vi "Smooth Volume.vi"(4 "Trigger":bool, 8 "Volume In":dbl format="%#_13g") -> (0 "Volume Out":sgl)   [LabVIEW 2015]
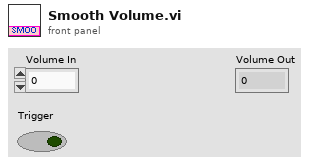
[diagram p1: front panel]
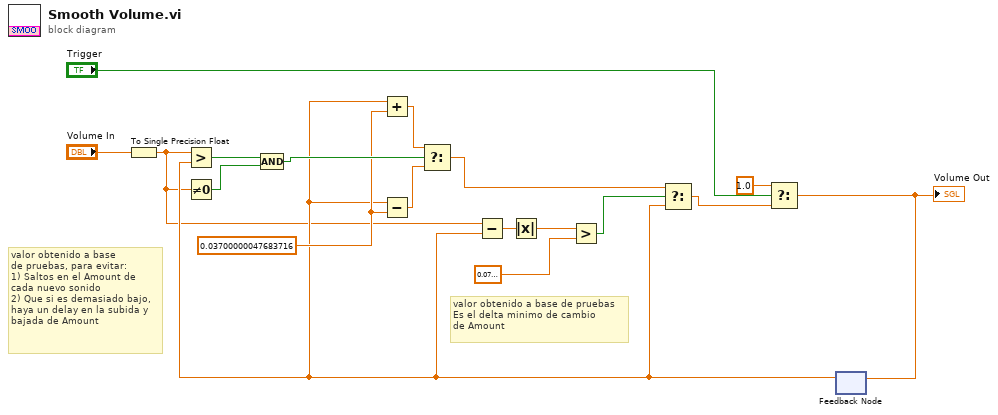
[diagram p0: block diagram]
diagram:
  w13 = sgl 0.037 ("factor")
  # "valor obtenido a base de pruebas\nEs el delta minimo de cambio\nde Amount"
  # "valor obtenido a base\nde pruebas, para evitar:\n1) Saltos en el Amount de\ncada nuevo sonido\n2) Que si es demasiado bajo,\nhaya un delay en la subida y\nbajada de Amount"
  n1 = To Single Precision Float(number="Volume In") -> (single precision float=w4:sgl)
  n2 = Not Equal To 0?(x=w4) -> (x != 0?=w14:bool)
  n3 = feedback #1() -> (w5:sgl)  [unwired: 1 in]
  n4 = Greater?(x=w4, y=w5) -> (0:w16:bool)
  n5 = Compound Arithmetic op=AND(w16, w14) -> (w15:bool)
  n6 = Add(x=w5, y=w13) -> (x+y=w17:sgl)
  n7 = Subtract(x=w5, y=w13) -> (x-y=w18:sgl)
  n8 = Select(t=w17, s=w15, f=w18) -> (s? t:f=w12:sgl)
  n9 = Subtract(x=w4, y=w5) -> (x-y=w11:sgl)
  n10 = Absolute Value(x=w11) -> (abs(x)=w10:sgl)
  n11 = Greater?(x=w10, y=sgl 0.07 ("tol")) -> (0:w9:bool)
  n12 = Select(t=w12, s=w9, f=w5) -> (s? t:f=w6:sgl)
  n13 = Select(t=sgl 1.0, s="Trigger", f=w6) -> (s? t:f=w1:sgl)
  "Volume Out" <- w1
  n14 = feedback-in #1(w1) -> ()
